vi "calculate deltaXbead.vi"(0 "X=T; Y=F":bool, 1 "Stage position (um)":dbl[](array[numeric]), 2 "QPD signal (V)":dbl[](array[numeric]), 3 "(1+2+3) stuckbead-scan coefficient":T1 {"(3)stuckbead-scan coefficient" min=0.0 max=127.0 format="%#.2f"; "(2)stuckbead-scan coefficient" min=0.0 max=127.0 format="%#.2f"; "(1)stuckbead-scan coefficient" min=0.0 max=127.0 format="%#.2f"}) -> (5 "delta Xbead (nm)":dbl[](array[numeric]), 7 "stage position out":dbl[](array[numeric]))   [LabVIEW 2014]
uses:
  (1+2+3)fit stuckbead coefficient.ctl
  <vilib>/Analysis/polynomials.llb/Scalar Polynomial Evaluation (DBL).vi
  <vilib>/Analysis/NI_AALPro.lvlib
panel:
  out "size(s) 2":i32
  out "size(s)":i32
  out "Waveform Chart":dbl[][](graph)
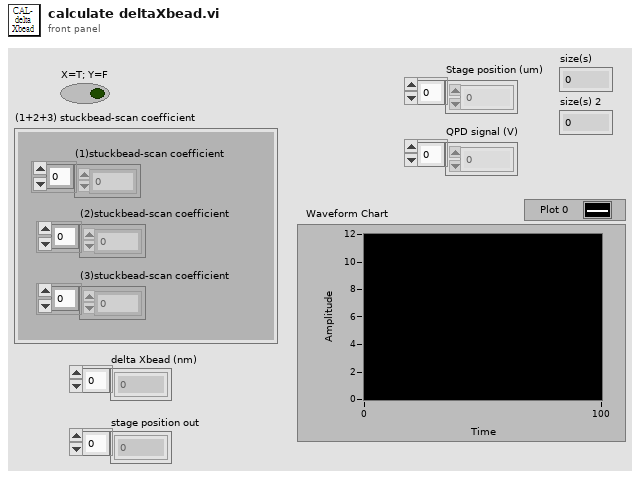
[diagram p1: front panel]
types:
  T1 = typedef "(1+2+3)fit stuckbead coefficient.ctl" = cluster{"(1)stuckbead-scan coefficient ":dbl[], "(2)stuckbead-scan coefficient ":dbl[], "(3)stuckbead-scan coefficient":dbl[]}
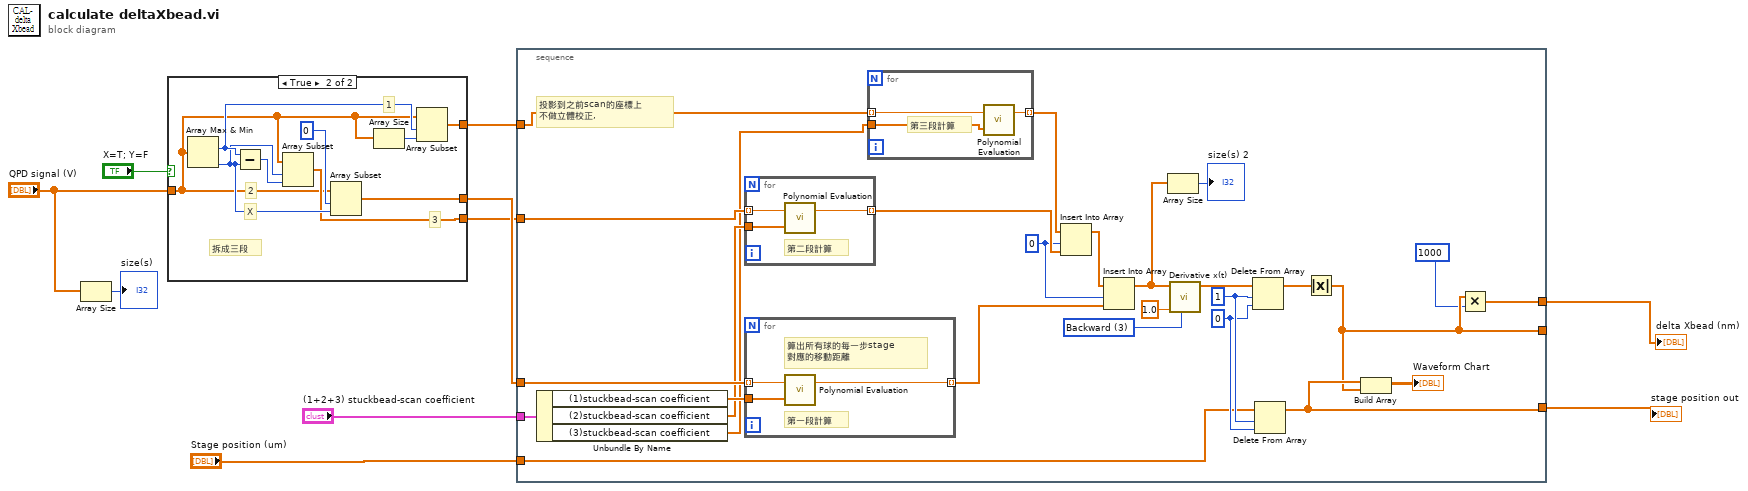
[diagram p0: block diagram]
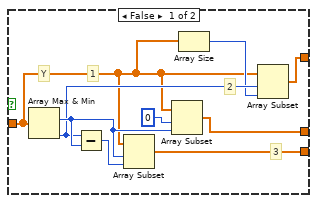
[diagram p2: hidden frame]
diagram:
  n1 = Array Size(array="QPD signal (V)") -> (size(s)=→"size(s)":i32)
  n2 = case shown="True" "X=T; Y=F" {
    tunnel: "QPD signal (V)" -> [w11 w20]
    tunnel: [w14 w23] -> w9
    tunnel: [w13 w22] -> w7
    tunnel: [w12 w21] -> w6
    frame False {
      # "Y"
      # "3"
      # "2"
      # "1"
      n3 = Array Max & Min(array=w11) -> (max index (indices)=w18:i32, min index (indices)=w16:i32)  [unwired: 2 out]
      n4 = Subtract(x=w16, y=w18) -> (x-y=w17:i32)
      n5 = Array Subset(array=w11, index=w18, length=w17) -> (w13:dbl[])
      n6 = Array Subset(array=w11, index=0, length=w18) -> (w14:dbl[])
      n7 = Array Size(array=w11) -> (size(s)=w15:i32)
      n8 = Array Subset(array=w11, index=w16, length=w15) -> (w12:dbl[])
    }
    frame True {
      # "拆成三段"
      # "X"
      # "3"
      # "2"
      # "1"
      n9 = Array Max & Min(array=w20) -> (max index (indices)=w26:i32, min index (indices)=w25:i32)  [unwired: 2 out]
      n10 = Subtract(x=w26, y=w25) -> (x-y=w24:i32)
      n11 = Array Subset(array=w20, index=w25, length=w24) -> (w22:dbl[])
      n12 = Array Subset(array=w20, index=0, length=w25) -> (w23:dbl[])
      n13 = Array Size(array=w20) -> (size(s)=w27:i32)
      n14 = Array Subset(array=w20, index=w26, length=w27) -> (w21:dbl[])
    }
  }
  n15 = stacked-sequence {
    tunnel: w9 -> [w54]
    tunnel: "(1+2+3) stuckbead-scan coefficient" -> [w53]
    tunnel: w7 -> [w50]
    tunnel: w6 -> [w48]
    tunnel: "Stage position (um)" -> [w35]
    tunnel: [w31] -> _
    tunnel: [w34] -> w4
    tunnel: [w29] -> w1
    frame #0 {
      w41 = 0 ("index")
      w36 = 0 ("index")
      w37 = 1 ("length")
      w46 = u16 3 items=["2nd Order Central", "4th Order Central", "Forward", "Backward"] ("method")
      # "投影到之前scan的座標上\n不做立體校正,"
      n16 = Unbundle By Name(w53) -> ("(1)stuckbead-scan coefficient"=w52:dbl[], "(2)stuckbead-scan coefficient"=w51:dbl[], "(3)stuckbead-scan coefficient"=w49:dbl[])
      n17 = for {
        tunnel: w50 -> [w60] mode=indexing
        tunnel: w51 -> [w59]
        tunnel: [w58] -> w42 mode=indexing
        # "第二段計算"
        n18 = call-poly <vilib>:"Polynomial Evaluation.vi"("P(x)"=w59, "a"=w60) -> ("P(a)"=w58:dbl)  [unwired: 1 out]
      }
      n19 = for {
        tunnel: w54 -> [w63] mode=indexing
        tunnel: w52 -> [w62]
        tunnel: [w61] -> w39 mode=indexing
        # "算出所有球的每一步stage\n對應的移動距離"
        # "第一段計算"
        n20 = call-poly <vilib>:"Polynomial Evaluation.vi"("P(x)"=w62, "a"=w63) -> ("P(a)"=w61:dbl)  [unwired: 1 out]
      }
      n21 = for {
        tunnel: w48 -> [w57] mode=indexing
        tunnel: w49 -> [w56]
        tunnel: [w55] -> w43 mode=indexing
        # "第三段計算"
        n22 = call-poly <vilib>:"Polynomial Evaluation.vi"("P(x)"=w56, "a"=w57) -> ("P(a)"=w55:dbl)  [unwired: 1 out]
      }
      n23 = Insert Into Array(array=w43, index=w41, new element=w42) -> (w40:dbl[])
      n24 = Insert Into Array(array=w40, index=w41, new element=w39) -> (w33:dbl[])
      n25 = Array Size(array=w33) -> (size(s)=→"size(s) 2":i32)
      n26 = call <vilib>:"Derivative x(t).vi"("method"=w46, "dt"=1.0, "X"=w33) -> ("dX/dt"=w45:dbl[])  [unwired: 7 in, 1 out]
      n27 = Delete From Array(array=w45, length=w37, index=w36) -> (array with subset deleted=w44:dbl[])  [unwired: 1 out]
      n28 = Delete From Array(array=w35, length=w37, index=w36) -> (array with subset deleted=w34:dbl[])  [unwired: 1 out]
      n29 = Absolute Value(x=w44) -> (abs(x)=w31:dbl[])
      n30 = Build Array(w34, w31) -> (→"Waveform Chart":dbl[][])
      n31 = Multiply(x=w31, y=1000) -> (x*y=w29:dbl[])
    }
  }
  "delta Xbead (nm)" <- w1
  "stage position out" <- w4
